vi "Open POP session.vi"(0 "username":string, 1 "password":string, 2 "POP server name/IP":string, 3 "error in":errorcluster) -> (5 "connection ID out":refnum<k5>, 7 "POP status":string, 8 "error out":errorcluster)   [LabVIEW 2012]
doc: "This VI opens a TCP/IP connection to a mail server machine using port 110, the standard POP TCP port.\n\nThe user is logged in with the password supplied, and the connection refnum is passed for subsequent communication."
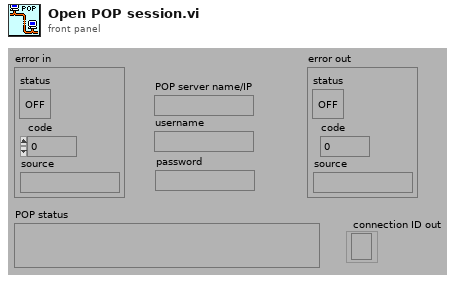
[diagram p1: front panel]
types:
  T1 = enum16{"Standard", "Buffered", "CRLF", "Immediate"}
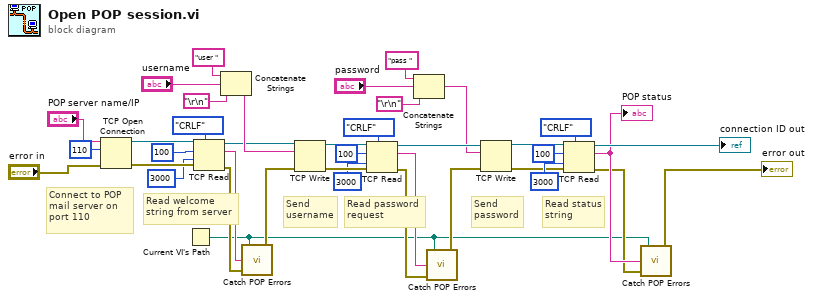
[diagram p0: block diagram]
diagram:
  # "Connect to POP\nmail server on\nport 110"
  # "Read status\nstring"
  # "Send\npassword"
  # "Read password\nrequest"
  # "Send\nusername"
  # "Read welcome\nstring from server"
  n1 = TCP Open Connection(address="POP server name/IP", remote port or service name=u16 110 ("remote port"), error in (no error)="error in") -> (connection ID=w27:refnum<k5>, error out=w26:errorcluster)  [unwired: 2 in]
  n2 = Current VI's Path() -> (path=w2:path)
  n3 = TCP Read(connection ID=w27, bytes to read=100, error in (no error)=w26, 7:T1."CRLF" ("mode (standard)"), 9:3000 ("timeout ms (25000)")) -> (connection ID out=w25:refnum<k5>, data out=w10:string, error out=w9:errorcluster)
  n4 = Concatenate Strings("user ", "username", "\r\n") -> (w34:string)
  n5 = call "Catch POP Errors.vi"("error in"=w9, "POP server response"=w10, "Caller Path"=w2) -> ("error out"=w8:errorcluster)
  n6 = TCP Write(connection ID=w25, data in=w34, error in (no error)=w8) -> (connection ID out=w32:refnum<k5>, error out=w31:errorcluster)  [unwired: 1 in, 1 out]
  n7 = TCP Read(connection ID=w32, bytes to read=100, error in (no error)=w31, 7:T1."CRLF" ("mode (standard)"), 9:3000 ("timeout ms (25000)")) -> (connection ID out=w19:refnum<k5>, data out=w7:string, error out=w6:errorcluster)
  n8 = Concatenate Strings("pass ", "password", "\r\n") -> (w18:string)
  n9 = call "Catch POP Errors.vi"("error in"=w6, "POP server response"=w7, "Caller Path"=w2) -> ("error out"=w5:errorcluster)
  n10 = TCP Write(connection ID=w19, data in=w18, error in (no error)=w5) -> (connection ID out=w14:refnum<k5>, error out=w13:errorcluster)  [unwired: 1 in, 1 out]
  n11 = TCP Read(connection ID=w14, bytes to read=100, error in (no error)=w13, 7:T1."CRLF" ("mode (standard)"), 9:3000 ("timeout ms (25000)")) -> (connection ID out=→"connection ID out":refnum<k5>, data out=w4:string, error out=w3:errorcluster)
  "POP status" <- w4
  n12 = call "Catch POP Errors.vi"("error in"=w3, "POP server response"=w4, "Caller Path"=w2) -> ("error out"=→"error out":errorcluster)
